vi "Launcher - New Worker.vi"() -> ()   [LabVIEW 2018]
uses:
  Workers/New Worker/Manager Worker.lvclass
  D:/Program Files (x86)/National Instruments/LabVIEW 2018/vi.lib/addons/_Workers/Library/Classes/Worker/Worker.lvclass
  Workers/New Worker/Initialization Data.ctl
  <vilib>/addons/_Workers/Debugger/Debug Client/Debug Client.lvlib
panel:
  out "error out":errorcluster
  in  "error in":errorcluster
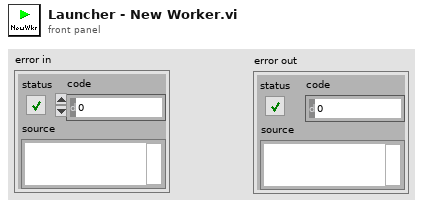
[diagram p1: front panel]
types:
  T1 = typedef "Manager Worker.lvclass/Initialization Data.ctl" = cluster{"String":string}
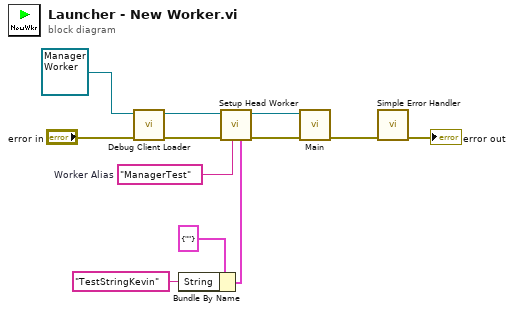
[diagram p0: block diagram]
diagram:
  w7 = "ManagerTest"  # Worker Alias
  n1 = call <vilib>:"Debug Client Loader.vi"("error in (no error)"="error in", "Worker"=refnum<class "Manager Worker.lvclass"> refnum ("Worker User Object")) -> ("error out"=w6:errorcluster, "Worker out"=w4:refnum<class "Manager Worker.lvclass">)  [unwired: 8 in]
  n2 = Bundle By Name(cluster=T1 {"String"=""} ("Initialization Data"), "String"="TestStringKevin") -> (w2:T1)
  n3 = call-dynamic "Setup Head Worker.vi"("Initalization Data"=w2, "Worker Alias"=w7, "error in"=w6, "Worker"=w4) -> ("error out"=w12:errorcluster, "Worker out"=w9:refnum<class "Manager Worker.lvclass">)  [unwired: 6 in]
  n4 = call-dynamic "Main.vi"("error in"=w12, "New Worker in"=w9) -> ("error out"=w10:errorcluster)  [unwired: 8 in, 1 out]
  n5 = call <vilib>:"Simple Error Handler.vi"("error in (no error)"=w10) -> ("error out"=→"error out":errorcluster)  [unwired: 4 in, 4 out]
